vi "MCL-Set Items Scroll To Last.vi"(0 "Multicolumn Listbox":refnum<vi>, 7 "Item Names":string[][](array[string]), 11 "error in (no error)":errorcluster) -> (15 "error out":errorcluster)   [LabVIEW 2020]
uses:
  <vilib>/Utility/miscctls.llb/LVRowAndColumnUnsignedTypeDef.ctl
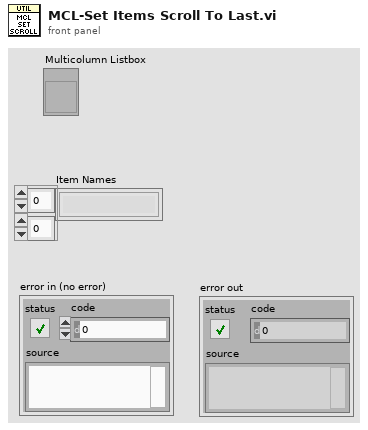
[diagram p1: front panel]
types:
  T1 = typedef "LVRowAndColumnUnsignedTypeDef.ctl" = cluster{"Row":u32, "Column":u32}
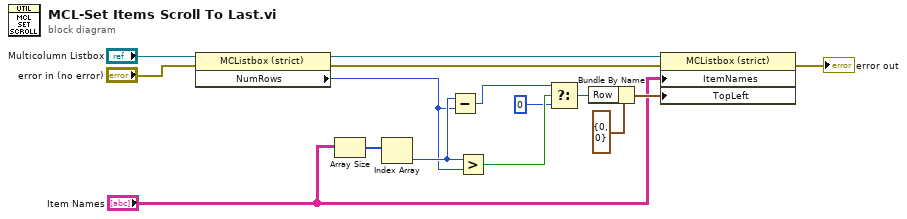
[diagram p0: block diagram]
diagram:
  n1 = property class="MCListbox (strict)"(reference="Multicolumn Listbox", error in="error in (no error)") -> (reference out=w2:refnum<vi>, error out=w1:errorcluster, "NumRows"=w8:u32)
  n2 = Array Size(array="Item Names") -> (size(s)=w15:i32[])
  n3 = Index Array(array=w15) -> (element=w12:i32)  [unwired: 1 in]
  n4 = Subtract(x=w12, y=w8) -> (x-y=w11:u32)
  n5 = Greater?(x=w12, y=w8) -> (0:w13:bool)
  n6 = Select(t=w11, s=w13, f=u32 0) -> (s? t:f=w9:u32)
  n7 = Bundle By Name(cluster=T1 {"Row"=0, "Column"=0} ("input cluster"), "Row"=w9) -> (w4:T1)
  n8 = property class="MCListbox (strict)"(reference=w2, error in=w1, "ItemNames"="Item Names", "TopLeft"=w4) -> (error out=→"error out":errorcluster)  [unwired: 1 out]
